vi "_34_Sample_qsns_9[10].vi"() -> ()   [LabVIEW 2020]
panel:
  out "Waveform Graph 2":i32[](graph)
  out "Array 2":i32[](array[numeric])
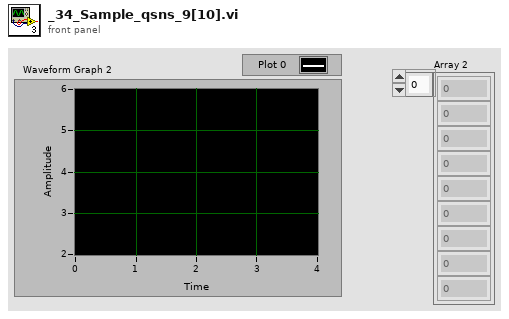
[diagram p1: front panel]
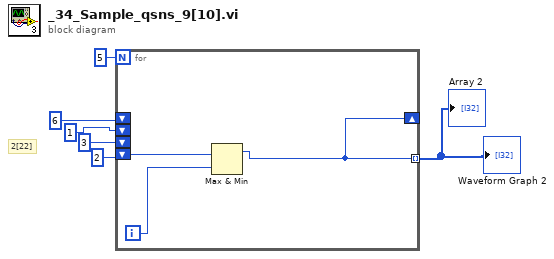
[diagram p0: block diagram]
diagram:
  # "2[22]"
  n1 = for {
    N: 5 -> [_]
    shift-right: [w7] -> _
    shift-left: 6 -> [_]
    shift-left: 1 -> [_]
    shift-left: 3 -> [_]
    shift-left: 2 -> [w9]
    tunnel: [w7] -> w1 mode=indexing
    i -> [w8]
    n2 = Max & Min(x=w9, y=w8) -> (max(x,y)=w7:i32)  [unwired: 1 out]
  }
  "Array 2" <- w1
  "Waveform Graph 2" <- w1
